vi "setSlitWidth.vi"(8 "error in (no error)":errorcluster, 10 "position":T2, 11 "MonoClientCommunicator in":refnum<class "MonoClientCommunicator.lvclass">) -> (0 "error out":errorcluster, 2 "ack":T1, 3 "MonoClientCommunicator out":refnum<class "MonoClientCommunicator.lvclass">)   [LabVIEW 2016, in "MonoClientCommunicator.lvclass"]
uses:
  MonoClientCommunicator.lvclass
  Typedefs/slit.ctl
  Typedefs/SlitType.ctl
  Typedefs/slitWidth.ctl
  Typedefs/AckType.ctl
  Typedefs/MonoCommand.ctl
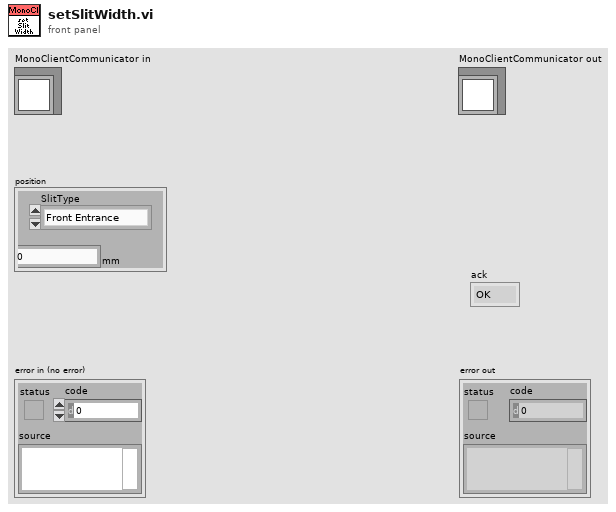
[diagram p1: front panel]
types:
  T1 = typedef "AckType.ctl" = enum16{"OK", "OutOfRange", "Unknown", "Busy", "Rejected"}
  T2 = typedef "slit.ctl" = cluster{"SlitType":T3, "Width":T4}
  T3 = typedef "SlitType.ctl" = enum16{"Front Entrance", "Side Entrance", "Front Exit", "Side Exit", "First Intermediate", "Second Intermediate"}
  T4 = typedef "slitWidth.ctl" = dbl[unit]
  T5 = typedef "MonoCommand.ctl" = enum16{"getGrating", "getFrontEntranceSlitPosition", "getFrontExitSlitPosition", "getWavelength", "setWavelength", "setGrating", "setFrontEntranceSlitPosition", "setFrontExitSlitPosition", "calibrateWavelength", "getStatus", "Unknown", "reset"}
  T6 = typedef "publishers.ctl" = enum16{"Wavelength", "Grating", "FrontEntranceSlitPosition", "FrontExitSlitPosition", "SoftwareStatus", "MonochromatorId", "Ack"}
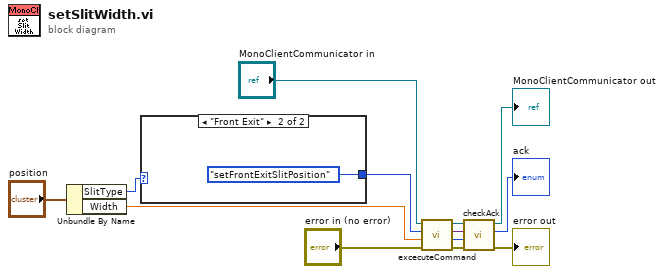
[diagram p0: block diagram]
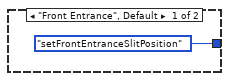
[diagram p2: hidden frame]
diagram:
  n1 = Unbundle By Name("position") -> ("SlitType"=w12:T3, "Width"=w3:T4)
  n2 = case shown="\"Front Exit\"" w12 {
    tunnel: [MonoCommand."setFrontEntranceSlitPosition" ("MonoCommand") MonoCommand."setFrontExitSlitPosition" ("MonoCommand")] -> w2
    frame "Front Entrance", Default {
    }
    frame "Front Exit" {
    }
  }
  n3 = call "excecuteCommand.vi"("error in (no error)"="error in (no error)", "input"=w3, "MonoCommand"=w2, "MonoClientCommunicator in"="MonoClientCommunicator in") -> ("error out"=w5:errorcluster, "parameter"=w6:T6, "value"=w7:variant, "MonoClientCommunicator out"=w8:refnum<class "MonoClientCommunicator.lvclass">)  [unwired: 4 in]
  n4 = call "checkAck.vi"("error in (no error)"=w5, "type"=w6, "value"=w7, "MonoClientCommunicator in"=w8) -> ("error out"=→"error out":errorcluster, "ack"=→"ack":T1, "MonoClientCommunicator out"=→"MonoClientCommunicator out":refnum<class "MonoClientCommunicator.lvclass">)  [unwired: 5 in]
